vi "Create Request.vi"(8 "error in (no error)":errorcluster, 9 "Notification? (F)":bool, 10 "params":variant, 11 "method":string) -> (0 "error out":errorcluster, 2 "{JSON} Requests":string, 3 "JSON-RPC out":refnum<class "JSON-RPC.lvclass">, 4 "ID":string)   [LabVIEW 2019, in "JSON-RPC.lvclass"]
uses:
  JSON-RPC.lvclass
  typedefs/Request--Cluster.ctl
  JSON-RPC.lvclass/JSON-RPC.ctl
  private/Create ID.vi
  private/Create Request-JSONtext.vi/6cd1d572-2af6-48e8-9b38-c51782860e23.vi
  private/Create Request-JSONtext.vi/7c5521bf-cb07-444f-843e-f9f289aa2aae.vi
  private/Create Request-JSONtext.vi/f6ae5555-b15c-4e52-b9b9-d6341c380ca9.vi
  private/Create Request-JSONtext.vi/6eedbf92-275d-42c0-90bb-b913601e88e9.vi
  <vilib>/Utility/Data Type/Get Type Information.vi
  <vilib>/JDP Science/JSONtext/Variant to JSON Text.vi
  <vilib>/JDP Science/JSONtext/Set Item.vi
  <vilib>/Utility/MD5Checksum.llb/MD5Checksum string.vi
  <vilib>/JDP Science/JSONtext/LVClass Serializer/JSONtext LVClass Serializer.lvclass
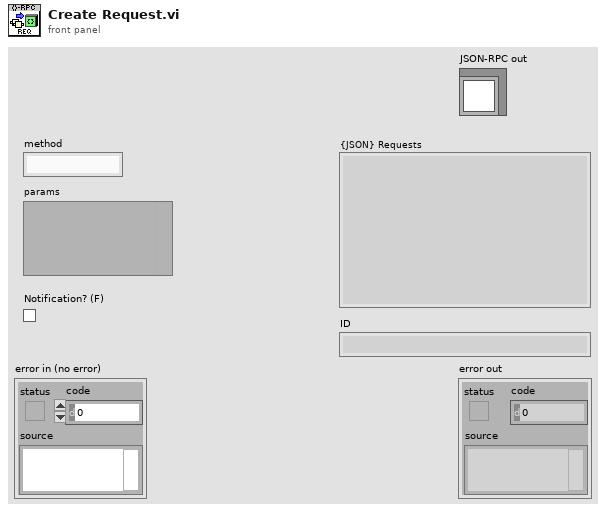
[diagram p1: front panel]
types:
  T1 = typedef "JSON-RPC.lvclass/Request--Cluster.ctl" = cluster{"method":string, "params":variant, "Notification?":bool}
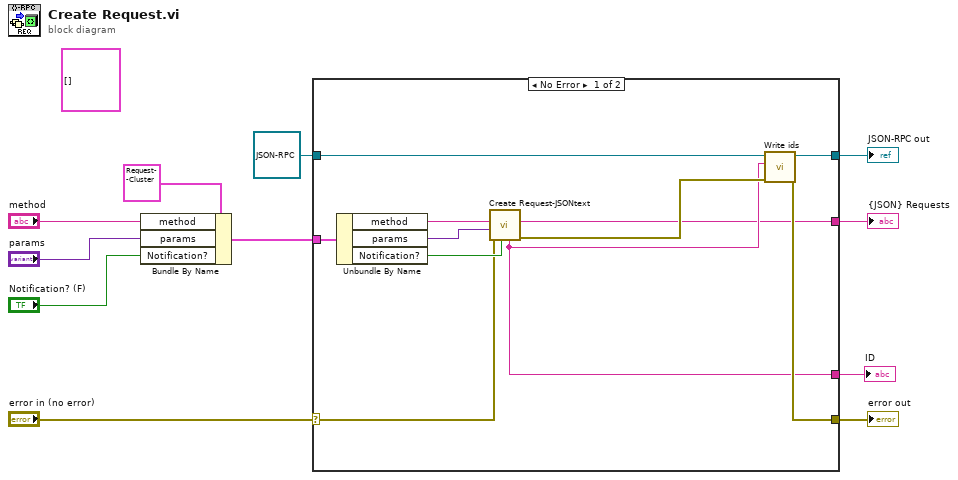
[diagram p0: block diagram]
diagram:
  (unwired) T1[] [] ("Requests")
  n1 = Bundle By Name(cluster=T1 {"method"="", "params"=variant, "Notification?"=FALSE} ("request"), "method"="method", "params"="params", "Notification?"="Notification? (F)") -> (w1:T1)
  n2 = case shown="No Error" "error in (no error)" {
    selector: "error in (no error)" -> [w14 w24]
    tunnel: [w21 w24] -> w10
    tunnel: [w20 w23] -> w8
    tunnel: refnum<class "JSON-RPC.lvclass"> refnum ("JSON-RPC in") -> [w19 w23]
    tunnel: [w12 _] -> w7
    tunnel: w1 -> [w22 _]
    tunnel: [w13 _] -> w6
    frame No Error {
      n3 = Unbundle By Name(w22) -> ("method"=w18:string, "params"=w17:variant, "Notification?"=w16:bool)
      n4 = call "Create Request-JSONtext.vi"("notification?"=w16, "error in (no error)"=w14, "params"=w17, "method"=w18) -> ("error out"=w15:errorcluster, "{JSON}"=w12:string, "id"=w13:string)  [unwired: 5 in]
      n5 = call "Write ids.vi"("error in (no error)"=w15, "ids"=w13, "JSON-RPC in"=w19) -> ("error out"=w21:errorcluster, "JSON-RPC out"=w20:refnum<class "JSON-RPC.lvclass">)  [unwired: 7 in]
    }
    frame Error {
    }
  }
  "error out" <- w10
  "JSON-RPC out" <- w8
  "{JSON} Requests" <- w7
  "ID" <- w6
